vi "Main.vi"(11 "Module Admin":refnum<class "Delacor_lib_QMH_Module Admin.lvclass">) -> ()   [LabVIEW 2024, in "Acquire.lvlib"]
doc: "This template is based off of the Queued Message Handler design pattern and the Queued Message Handler project template that ships with LabVIEW.\n\nThe main difference is that the queue is private to this module and communication between modules is performed via Broadcast and Request events.\n\nRequest events are wrapped in public API methods and are handled in the Event Handling Loop (EHL) of this VI. Any module can register for Broadcast events sent by this module. The EHL generates messages based on user interface actions.\n\nThe Message Handling Loop (MHL) processes messages generated by the EHL, or by other messages. The messages are string values, so new messages can be added easily to the Message Cases case structure in the MHL. Each message cluster can also provide an optional value for Message Data, which is a variant that can be converted to whatever message-specific data is required.\n_____\nBased on DQMH Project Template 7.0.1.1316."
uses:
  Acquire.lvlib
  <vilib>/Delacor/Delacor QMH/Libraries/Module Admin_class/Delacor_lib_QMH_Module Admin.lvclass
  Module Data--cluster.ctl
  <vilib>/Delacor/Delacor QMH/Libraries/Message Queue_class/Delacor_lib_QMH_Message Queue.lvclass/Delacor_lib_QMH_Message Queue.ctl
  Stop Argument--cluster.ctl
  <vilib>/Delacor/Delacor QMH/Libraries/Module Admin_class/Delacor_lib_QMH_Module Admin.lvclass/Delacor_lib_QMH_Module Admin.ctl
  Data Received Argument--cluster.ctl
  Start Recording Argument--cluster.ctl
  Stop Recording Argument--cluster.ctl
  Start Acquisition Argument--cluster.ctl
  Stop Acquisition Argument--cluster.ctl
  Get Reference Argument--cluster.ctl
  Get Reference (Reply Payload)--cluster.ctl
  DAQ/DAQ Config.ctl
  <vilib>/Delacor/Delacor QMH/Libraries/Message Queue_class/Delacor_lib_QMH_Enqueue Message (Single).vi
  <vilib>/Delacor/Delacor QMH/Libraries/Module Admin_class/Delacor_lib_QMH_Get External Launch.vi
  <vilib>/Delacor/Delacor QMH/Libraries/Message Queue_class/Delacor_lib_QMH_Message Queue.lvclass
  DAQ/DAQ.lvlib
panel:
  out "Waveform Chart":waveform(dbl)[](graph)
  in  "Acquire":bool
  in  "Record":bool
  out "error out":errorcluster
  out "Status":string
  in  "Simulate MHL Error":bool
  in  "Simulate EHL Error":bool
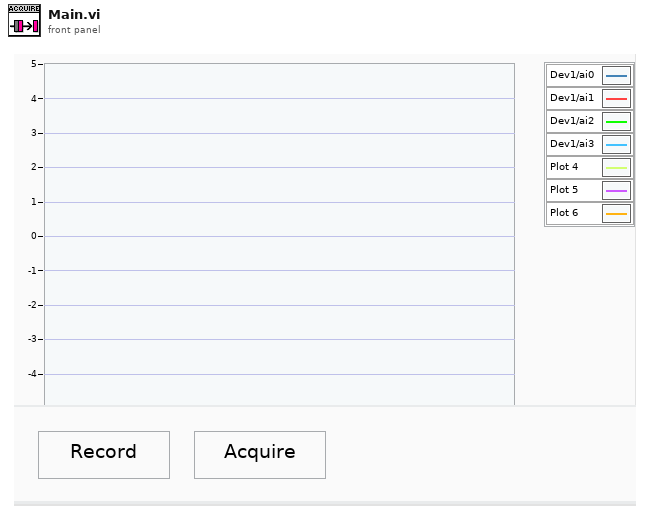
[diagram p1: front panel]
types:
  T1 = typedef "Acquire.lvlib/Request Events--cluster.ctl" = cluster{"Stop Module":refnum<user-event>, "Show Panel":refnum<user-event>, "Hide Panel":refnum<user-event>, "Get Module Execution Status":refnum<user-event>, "Show Diagram":refnum<user-event>, "Private":cluster{"Data Received":refnum<user-event>}, "Start Recording":refnum<user-event>, "Stop Recording":refnum<user-event>, "Start Acquisition":refnum<user-event>, "Stop Acquisition":refnum<user-event>, "Get Reference":refnum<user-event>}
  T2 = typedef "DAQ.lvlib/Broadcast Events--cluster.ctl" = cluster{"Module Did Init":refnum<user-event>, "Status Updated":refnum<user-event>, "Error Reported":refnum<user-event>, "Module Did Stop":refnum<user-event>, "Update Module Execution Status":refnum<user-event>, "New Data":refnum<user-event>}
  T3 = typedef "Acquire.lvlib/Module Data--cluster.ctl" = cluster{"Status":string, "Recording?":bool, "tdms file out":refnum<k34>, "Acquiring?":bool}
  T4 = enum32{"invalid lock state", "Not Locked", "Locked (No Password)", "Password-protected"}
  T5 = typedef "Acquire.lvlib/Stop Argument--cluster.ctl" = cluster{"Origin":string, "Exit via Stop Module Req?":bool, "Wait for Module to stop?":bool}
  T6 = typedef "Acquire.lvlib/Data Received Argument--cluster.ctl" = cluster{"Data":waveform(dbl)[]}
  T7 = typedef "Acquire.lvlib/Start Recording Argument--cluster.ctl" = cluster{"File Path":path}
  T8 = typedef "Acquire.lvlib/Stop Recording Argument--cluster.ctl" = cluster{"Boolean":bool}
  T9 = typedef "Acquire.lvlib/Start Acquisition Argument--cluster.ctl" = cluster{"Boolean":bool}
  T10 = typedef "Acquire.lvlib/Stop Acquisition Argument--cluster.ctl" = cluster{"Boolean":bool}
  T11 = typedef "Acquire.lvlib/Get Reference Argument--cluster.ctl" = cluster{"Wait Notifier":refnum<notifier>, "wait for reply":bool}
  T12 = enum32{"Invalid", "Standard", "Closed", "Hidden", "Minimized", "Maximized"}
  T13 = enum16{"open", "open or create", "create or replace", "create", "open (read-only)"}
  T14 = typedef "DAQ.lvlib/DAQ Config.ctl" = cluster{"DAQmx Channel":tag, "Samplerate":dbl, "# Samples":i32}
  T15 = typedef "Acquire.lvlib/Get Reference (Reply Payload)--cluster.ctl" = cluster{"Main VI":refnum<vi>, "error":errorcluster}
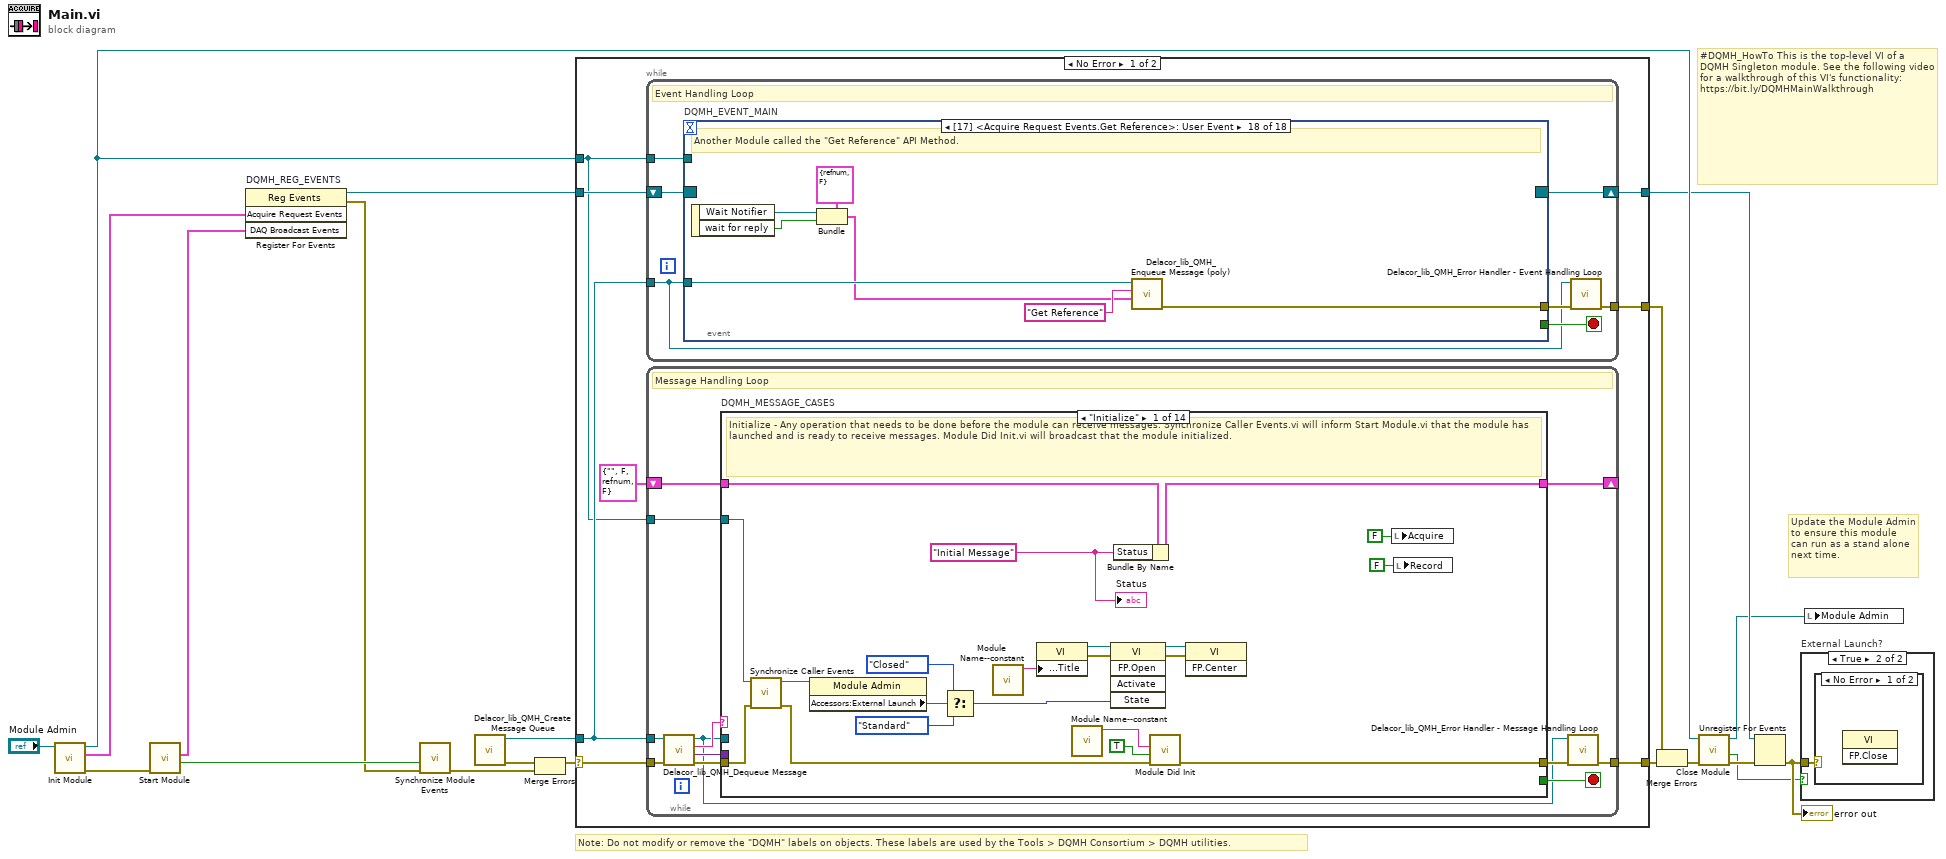
[diagram p0: block diagram]
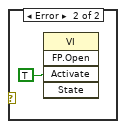
[diagram p3: hidden frame]
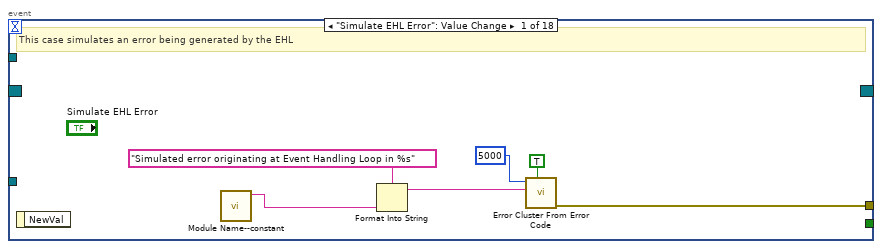
[diagram p4: hidden frame]
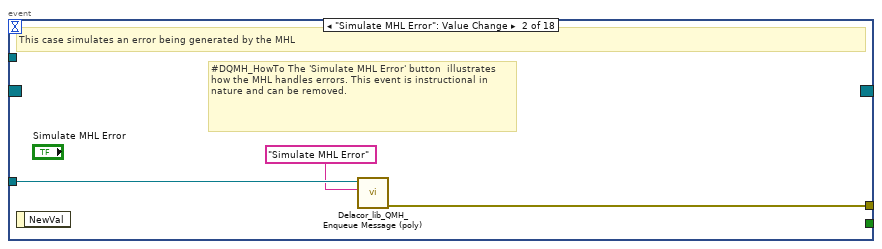
[diagram p5: hidden frame]
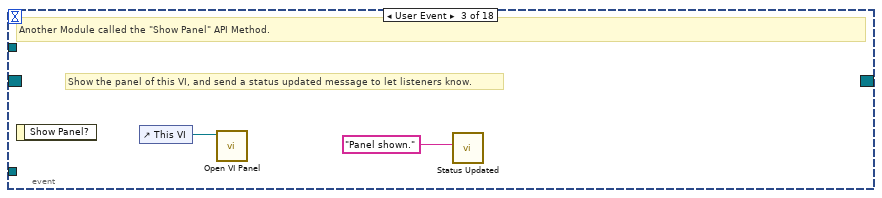
[diagram p6: hidden frame]
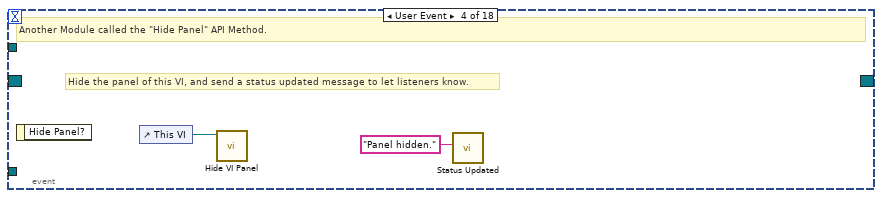
[diagram p7: hidden frame]
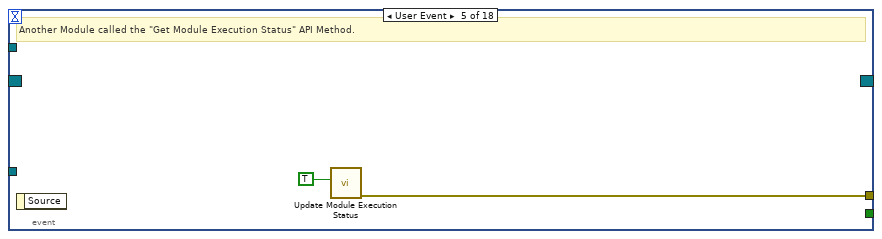
[diagram p8: hidden frame]
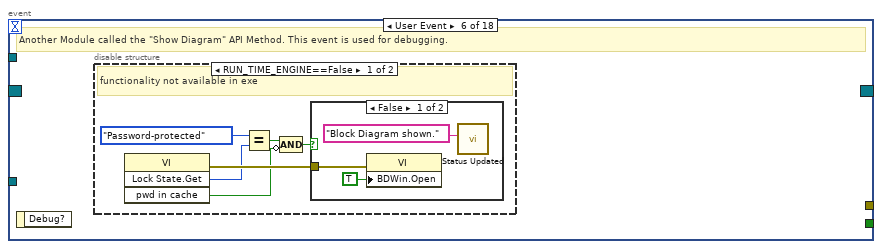
[diagram p9: hidden frame]
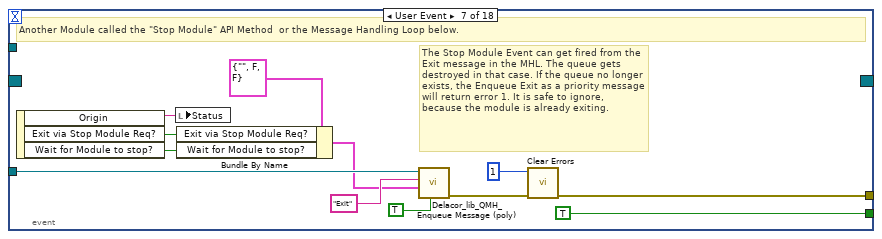
[diagram p12: hidden frame]
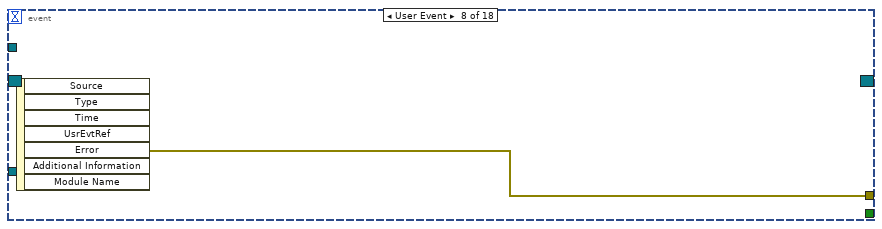
[diagram p13: hidden frame]
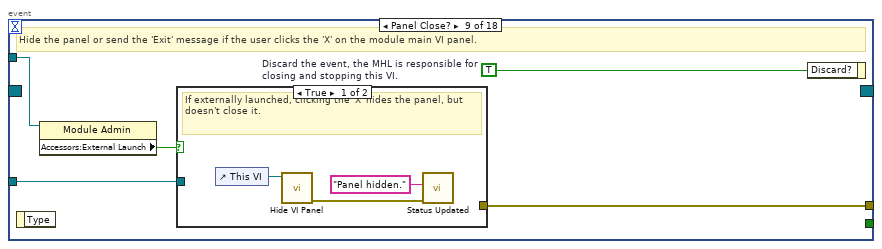
[diagram p14: hidden frame]
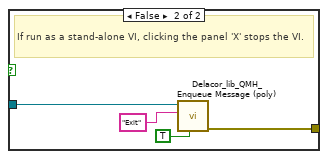
[diagram p15: hidden frame]
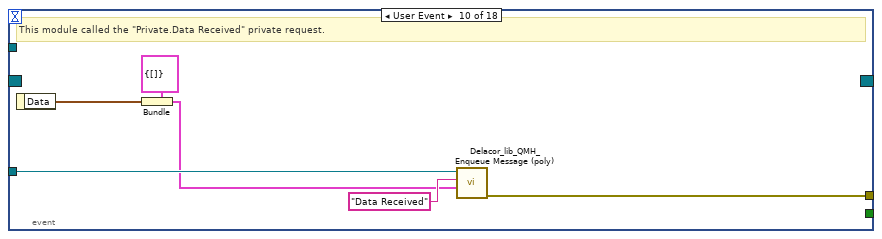
[diagram p16: hidden frame]
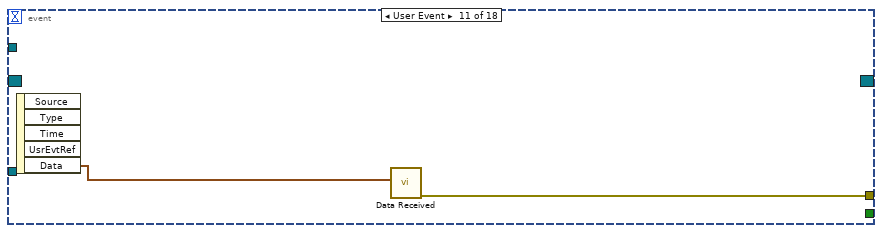
[diagram p17: hidden frame]
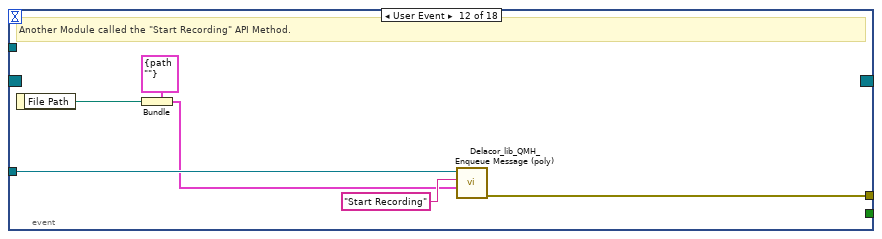
[diagram p18: hidden frame]
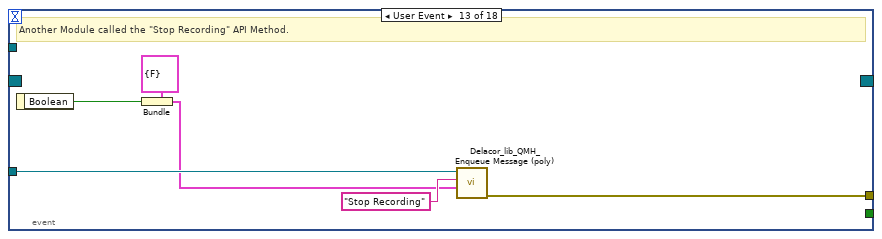
[diagram p19: hidden frame]
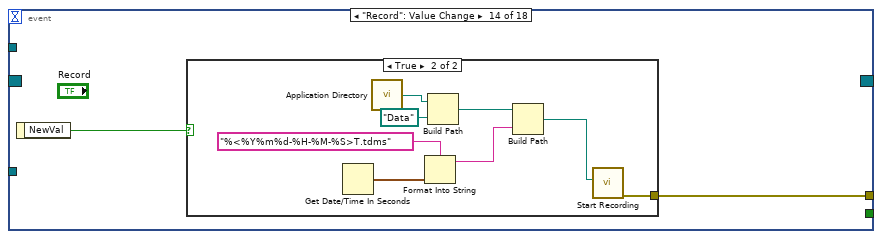
[diagram p20: hidden frame]
diagram:
  # "#DQMH_HowTo This is the top-level VI of a DQMH Singleton module. See the following video for a walkthrough of this VI's functionality: https://bit.ly/DQMHMainWalkthrough"
  # "Note: Do not modify or remove the \"DQMH\" labels on objects. These labels are used by the Tools > DQMH Consortium > DQMH utilities."
  # "Update the Module Admin to ensure this module can run as a stand alone next time."
  n1 = call "Init Module.vi"("Singleton Module Admin in"="Module Admin") -> ("error out"=w19:errorcluster, "Acquire Request Events"=w9:T1, "Singleton Module Admin out"=w12:refnum<class "Delacor_lib_QMH_Module Admin.lvclass">)  [unwired: 8 in]
  n2 = call "Start Module.vi"("error in"=w19) -> ("Wait for Event Sync?"=w3:bool, "DAQ Broadcast Events"=w4:T2)  [unwired: 7 in, 2 out]
  n3 = register-events "DQMH_REG_EVENTS"(w9, w4) -> (reference out=w10:refnum<event-registration>, error out=w2:errorcluster)  [unwired: 2 in]
  n4 = call "Synchronize Module Events.vi"("error in"=w2, "Wait for Event Sync?"=w3) -> ("error out"=w1:errorcluster)  [unwired: 9 in]
  n5 = call <vilib>:"Delacor_lib_QMH_Create Message Queue.vi"() -> ("error out"=w14:errorcluster, "Message Queue"=w8:refnum<class "Delacor_lib_QMH_Message Queue.lvclass">)  [unwired: 10 in]
  n6 = Merge Errors(w14, w1) -> (w13:errorcluster)
  n7 = case shown="No Error" w13 {
    selector: w13 -> [w26 w332]
    tunnel: [w28 w331] -> w20
    tunnel: [w25 w330] -> w11
    tunnel: w10 -> [w23 w330]
    tunnel: w8 -> [w22 w325]
    tunnel: [w27 _] -> w17
    tunnel: w12 -> [w21 w326]
    frame No Error {
      n8 = while {
        tunnel: w22 -> [w29]
        shift-right: [w32] -> w25
        shift-left: w23 -> [w33]
        tunnel: [w34] -> w27
        tunnel: w21 -> [w30]
        stop <- w31 stop-if-true
        # "Event Handling Loop"
        n9 = event "DQMH_EVENT_MAIN" shown="[17] <Acquire Request Events.Get Reference>: User Event" {
          selector: w33 -> [_ _ _ _ _ _ _ _ _ _ _ _ _ _ _ _ _ _]
          dyn-events: [_ _ _ _ _ _ _ _ _ _ _ _ _ _ _ _ _ _] -> w32
          timeout: _ -> [_ _ _ _ _ _ _ _ _ _ _ _ _ _ _ _ _ _]
          tunnel: [_ _ _ _ _ _ TRUE ("Discard?") _ _ _ _ _ _ _ _ _ _ _] -> w31
          tunnel: w29 -> [_ w43 _ _ _ _ w67 _ w75 w90 _ w98 w104 _ _ w125 w131 w138]
          tunnel: [w41 w44 _ _ w50 _ w70 w72 w77 w85 w91 w93 w99 w105 w117 w120 w126 w132] -> w35
          tunnel: w30 -> [_ _ _ _ _ _ _ _ w74 _ _ _ _ _ _ _ _ _]
          event "Simulate EHL Error": Value Change {
            # "This case simulates an error being generated by the EHL"
            n10 = event-data() -> ()  [unwired: 1 in, 1 out]
            n11 = call "Module Name--constant.vi"() -> ("Module Name"=w38:string)  [unwired: 11 in]
            n12 = Format Into String(format string="Simulated error originating at Event Handling Loop in %s", w38) -> (resulting string=w39:string)  [unwired: 2 in, 1 out]
            n13 = call <vilib>:"Error Cluster From Error Code.vi"("show call chain? (False)"=TRUE, "error message (\"\")"=w39, "error code (0)"=5000) -> ("error out"=w41:errorcluster)  [unwired: 6 in]
          }
          event "Simulate MHL Error": Value Change {
            # "#DQMH_HowTo The 'Simulate MHL Error' button  illustrates how the MHL handles errors. This event is instructional in nature and can be removed."
            # "This case simulates an error being generated by the MHL"
            n14 = event-data() -> ()  [unwired: 1 in, 1 out]
            n15 = call-poly <vilib>:"Delacor_lib_QMH_Enqueue Message (poly).vi"("Message"="Simulate MHL Error", "Message Queue in"=w43) -> ("error out"=w44:errorcluster)  [unwired: 8 in, 1 out]
          }
          event User Event {
            # "Show the panel of this VI, and send a status updated message to let listeners know."
            # "Another Module called the \"Show Panel\" API Method."
            n16 = event-data() -> ()  [unwired: 1 in, 1 out]
            n17 = control-ref of="This VI"() -> (w46:refnum<vi>)
            n18 = call "Open VI Panel.vi"("VI"=w46) -> ()  [unwired: 10 in, 1 out]
            n19 = call "Status Updated.vi"("Status"="Panel shown." ("format string")) -> ()  [unwired: 10 in, 1 out]
          }
          event User Event {
            # "Hide the panel of this VI, and send a status updated message to let listeners know."
            # "Another Module called the \"Hide Panel\" API Method."
            n20 = event-data() -> ()  [unwired: 1 in, 1 out]
            n21 = control-ref of="This VI"() -> (w48:refnum<vi>)
            n22 = call "Hide VI Panel.vi"("VI"=w48) -> ()  [unwired: 10 in, 1 out]
            n23 = call "Status Updated.vi"("Status"="Panel hidden." ("format string")) -> ()  [unwired: 10 in, 1 out]
          }
          event User Event {
            # "Another Module called the \"Get Module Execution Status\" API Method."
            n24 = event-data() -> ()  [unwired: 1 in, 1 out]
            n25 = call "Update Module Execution Status.vi"("Running?"=TRUE) -> ("error out"=w50:errorcluster)  [unwired: 10 in]
          }
          event User Event {
            # "Another Module called the \"Show Diagram\" API Method. This event is used for debugging."
            n26 = event-data() -> ()  [unwired: 1 in, 1 out]
            n27 = disable-structure shown="RUN_TIME_ENGINE==False" {
              frame condition #0 (active) {
                # "functionality not available in exe"
                n28 = invoke on="Invoke Node" class="VI" method="Lock State.Get"() -> (error out=w56:errorcluster, "Get Lock State"=w55:T4, "pwd in cache"=w52:bool)  [unwired: 4 in, 1 out]
                n29 = Equal?(x=T4."Password-protected", y=w55) -> (x = y?=w53:bool)
                n30 = Compound Arithmetic op=AND(w53, invert w52) -> (w51:bool)
                n31 = case shown="False" w51 {
                  tunnel: w56 -> [w59 _]
                  frame False {
                    n32 = property on="Property Node" class="VI"(error in=w59, "BDWin.Open"=TRUE ("Block Diagram Window:Open")) -> ()  [unwired: 1 in, 2 out]
                    n33 = call "Status Updated.vi"("Status"="Block Diagram shown." ("format string")) -> ()  [unwired: 10 in, 1 out]
                  }
                  frame True {
                    # "Password-protected VI, and the password is not in the cache. Do not show the diagram."
                  }
                }
              }
              frame condition #1 {
              }
            }
          }
          event User Event {
            # "The Stop Module Event can get fired from the Exit message in the MHL. The queue gets destroyed in that case. If the queue no longer exists, the Enqueue Exit as a priority message will return error 1. It is safe to ignore, because the module is already exiting."
            # "Another Module called the \"Stop Module\" API Method  or the Message Handling Loop below."
            n34 = event-data() -> ("Origin"=w66:string, "Exit via Stop Module Req?"=w62:bool, "Wait for Module to stop?"=w61:bool)  [unwired: 1 in]
            n35 = local write "Status"(w66) -> ()
            n36 = Bundle By Name(cluster=T5 {"Origin"="", "Exit via Stop Module Req?"=FALSE, "Wait for Module to stop?"=FALSE} ("Stop Argument"), "Exit via Stop Module Req?"=w62, "Wait for Module to stop?"=w61) -> (w60:T5)
            n37 = call-poly <vilib>:"Delacor_lib_QMH_Enqueue Message (poly).vi"("Priority Message? (F)"=TRUE, "Message Data"=w60, "Message"="Exit", "Message Queue in"=w67) -> ("error out"=w71:errorcluster)  [unwired: 6 in, 1 out]
            n38 = call <vilib>:"Clear Errors.vi"("error in (no error)"=w71, "specific error code to clear (0: all)"=1) -> ("error out"=w70:errorcluster)  [unwired: 4 in, 1 out]
          }
          event User Event {
            n39 = event-data() -> ("Error"=w72:errorcluster)  [unwired: 1 in, 6 out]
          }
          event Panel Close? {
            w76 = TRUE  # Discard the event, the MHL is responsible for closing and stopping this VI.
            # "Hide the panel or send the 'Exit' message if the user clicks the 'X' on the module main VI panel."
            n40 = event-data() -> ()  [unwired: 1 in, 1 out]
            n41 = property on="Property Node" class="Module Admin"(reference=w74) -> ("Accessors:External Launch"=w73:bool)  [unwired: 1 in, 2 out]
            n42 = case shown="True" w73 {
              tunnel: w75 -> [_ w83]
              tunnel: [_ w84] -> w77
              frame True {
                # "If externally launched, clicking the 'X' hides the panel, but doesn't close it."
                n43 = control-ref of="This VI"() -> (w80:refnum<vi>)
                n44 = call "Hide VI Panel.vi"("VI"=w80) -> ("error out"=w78:errorcluster)  [unwired: 10 in]
                n45 = call "Status Updated.vi"("error in"=w78, "Status"="Panel hidden." ("format string")) -> ()  [unwired: 9 in, 1 out]
              }
              frame False {
                # "If run as a stand-alone VI, clicking the panel 'X' stops the VI."
                n46 = call-poly <vilib>:"Delacor_lib_QMH_Enqueue Message (poly).vi"("Priority Message? (F)"=TRUE, "Message"="Exit", "Message Queue in"=w83) -> ("error out"=w84:errorcluster)  [unwired: 7 in, 1 out]
              }
            }
            n47 = event-data ("Event Filter Node")("Discard?"=w76) -> ()  [unwired: 1 in, 1 out]
          }
          event User Event {
            # "This module called the \"Private.Data Received\" private request."
            n48 = event-data() -> ("Data"=w86:waveform(dbl)[])  [unwired: 1 in]
            n49 = Bundle(cluster=T6 {"Data"=[]} ("Data Received Argument"), "Data"=w86) -> (w87:T6)
            n50 = call-poly <vilib>:"Delacor_lib_QMH_Enqueue Message (poly).vi"("Message Data"=w87, "Message"="Data Received", "Message Queue in"=w90) -> ("error out"=w85:errorcluster)  [unwired: 7 in, 1 out]
          }
          event User Event {
            n51 = event-data() -> ("Data"=w92:waveform(dbl)[])  [unwired: 1 in, 4 out]
            n52 = call "Data Received.vi"("Data"=w92) -> ("error out"=w91:errorcluster)  [unwired: 10 in]
          }
          event User Event {
            # "Another Module called the \"Start Recording\" API Method."
            n53 = event-data() -> ("File Path"=w94:path)  [unwired: 1 in]
            n54 = Bundle(cluster=T7 {"File Path"=path ""} ("Start Recording Argument"), "File Path"=w94) -> (w95:T7)
            n55 = call-poly <vilib>:"Delacor_lib_QMH_Enqueue Message (poly).vi"("Message Data"=w95, "Message"="Start Recording", "Message Queue in"=w98) -> ("error out"=w93:errorcluster)  [unwired: 7 in, 1 out]
          }
          event User Event {
            # "Another Module called the \"Stop Recording\" API Method."
            n56 = event-data() -> ("Boolean"=w100:bool)  [unwired: 1 in]
            n57 = Bundle(cluster=T8 {"Boolean"=FALSE} ("Stop Recording Argument"), "Boolean"=w100) -> (w101:T8)
            n58 = call-poly <vilib>:"Delacor_lib_QMH_Enqueue Message (poly).vi"("Message Data"=w101, "Message"="Stop Recording", "Message Queue in"=w104) -> ("error out"=w99:errorcluster)  [unwired: 7 in, 1 out]
          }
          event "Record": Value Change {
            n59 = event-data() -> ("NewVal"=w106:bool)  [unwired: 1 in]
            n60 = case shown="True" w106 {
              tunnel: [w107 w115] -> w105
              frame False {
                n61 = call "Stop Recording.vi"() -> ("error out"=w107:errorcluster)  [unwired: 11 in]
              }
              frame True {
                n62 = Get Date/Time In Seconds() -> (seconds since 1Jan1904=w112:timestamp)
                n63 = call <vilib>:"Application Directory.vi"() -> ("Application Directory"=w109:path)
                n64 = Format Into String(format string="%<%Y%m%d-%H-%M-%S>T.tdms", w112) -> (resulting string=w114:string)  [unwired: 2 in, 1 out]
                n65 = Build Path(base path=w109, name or relative path=path "Data") -> (appended path=w111:path)
                n66 = Build Path(base path=w111, name or relative path=w114) -> (appended path=w108:path)
                n67 = call "Start Recording.vi"("File Path"=w108) -> ("error out"=w115:errorcluster)  [unwired: 10 in]
              }
            }
          }
          event "Acquire": Value Change {
            n68 = event-data() -> ("NewVal"=w116:bool)  [unwired: 1 in]
            n69 = case shown="True" w116 {
              tunnel: [w118 w119] -> w117
              frame False {
                n70 = call "Stop Acquisition.vi"() -> ("error out"=w118:errorcluster)  [unwired: 11 in]
              }
              frame True {
                n71 = call "Start Acquisition.vi"() -> ("error out"=w119:errorcluster)  [unwired: 11 in]
              }
            }
          }
          event User Event {
            # "Another Module called the \"Start Acquisition\" API Method."
            n72 = event-data() -> ("Boolean"=w121:bool)  [unwired: 1 in]
            n73 = Bundle(cluster=T9 {"Boolean"=FALSE} ("Start Acquisition Argument"), "Boolean"=w121) -> (w122:T9)
            n74 = call-poly <vilib>:"Delacor_lib_QMH_Enqueue Message (poly).vi"("Message Data"=w122, "Message"="Start Acquisition", "Message Queue in"=w125) -> ("error out"=w120:errorcluster)  [unwired: 7 in, 1 out]
          }
          event User Event {
            # "Another Module called the \"Stop Acquisition\" API Method."
            n75 = event-data() -> ("Boolean"=w127:bool)  [unwired: 1 in]
            n76 = Bundle(cluster=T10 {"Boolean"=FALSE} ("Stop Acquisition Argument"), "Boolean"=w127) -> (w128:T10)
            n77 = call-poly <vilib>:"Delacor_lib_QMH_Enqueue Message (poly).vi"("Message Data"=w128, "Message"="Stop Acquisition", "Message Queue in"=w131) -> ("error out"=w126:errorcluster)  [unwired: 7 in, 1 out]
          }
          event User Event {
            # "Another Module called the \"Get Reference\" API Method."
            n78 = event-data() -> ("Wait Notifier"=w134:refnum<notifier>, "wait for reply"=w133:bool)  [unwired: 1 in]
            n79 = Bundle(cluster=T11 {"Wait Notifier"=refnum, "wait for reply"=FALSE} ("Get Reference Argument"), "Wait Notifier"=w134, "wait for reply"=w133) -> (w135:T11)
            n80 = call-poly <vilib>:"Delacor_lib_QMH_Enqueue Message (poly).vi"("Message Data"=w135, "Message"="Get Reference", "Message Queue in"=w138) -> ("error out"=w132:errorcluster)  [unwired: 7 in, 1 out]
          }
        }
        n81 = call-dynamic "Delacor_lib_QMH_Error Handler - Event Handling Loop.vi"("error in"=w35, "Message Queue in"=w29) -> ("dup error in"=w34:errorcluster)  [unwired: 8 in, 1 out]
      }
      n82 = while {
        tunnel: w22 -> [w139]
        shift-right: [w147] -> _
        shift-left: T3 {"Status"="", "Recording?"=FALSE, "tdms file out"=refnum, "Acquiring?"=FALSE} ("Data Cluster") -> [w148]
        tunnel: w26 -> [w150]
        tunnel: [w142] -> w28
        tunnel: w21 -> [w143]
        stop <- w146 stop-if-true
        # "Message Handling Loop"
        n83 = call-dynamic "Delacor_lib_QMH_Dequeue Message.vi"("error in"=w150, "Message Queue in"=w139) -> ("error out"=w149:errorcluster, "Message Data"=w144:variant, "Message"=w145:string, "Message Queue out"=w140:refnum<class "Delacor_lib_QMH_Message Queue.lvclass">)  [unwired: 6 in]
        n84 = case "DQMH_MESSAGE_CASES" shown="\"Initialize\"" w145 {
          selector: w145 -> [_ _ _ _ _ _ _ _ _ _ _ _ _ w320]
          tunnel: w140 -> [_ _ _ _ _ _ _ _ _ _ _ w285 w308 _]
          tunnel: w149 -> [w169 w173 w185 w204 w231 w244 w252 w265 w270 w272 w281 w292 w314 w323]
          tunnel: [w167 w173 w180 w198 w229 w245 w251 w255 w269 w272 w280 w288 w309 w324] -> w141
          tunnel: w148 -> [w158 w172 w178 w196 w228 w248 w253 w264 w268 w271 w278 w287 w307 w321]
          tunnel: [w157 w172 w177 w199 w230 w243 w250 w264 w268 w271 w278 w287 w307 w321] -> w147
          tunnel: [_ _ _ _ _ _ _ _ _ _ _ _ w306 _] -> w146
          tunnel: w144 -> [_ _ w183 w202 _ _ _ w262 _ _ _ w286 w305 _]
          tunnel: w143 -> [w159 _ _ _ _ _ _ _ _ _ _ w284 w300 _]
          frame "Initialize" {
            w153 = "Initial Message" ("Initial Message")
            # "Initialize - Any operation that needs to be done before the module can receive messages. Synchronize Caller Events.vi will inform Start Module.vi that the module has launched and is ready to receive messages. Module Did Init.vi will broadcast that the module initialized."
            n85 = call "Synchronize Caller Events.vi"("error in"=w169, "Singleton Module Admin in"=w159) -> ("error out"=w168:errorcluster, "Singleton Module Admin out"=w154:refnum<class "Delacor_lib_QMH_Module Admin.lvclass">)  [unwired: 8 in]
            n86 = property on="Property Node" class="Module Admin"(reference=w154) -> ("Accessors:External Launch"=w163:bool)  [unwired: 1 in, 2 out]
            n87 = Select(t=T12."Closed" ("State"), s=w163, f=T12."Standard" ("State")) -> (s? t:f=w160:T12)
            n88 = call "Module Name--constant.vi"() -> ("Module Name"=w166:string)  [unwired: 11 in]
            n89 = property on="Property Node" class="VI"("Front Panel.Title"=w166) -> (reference out=w165:refnum<vi>, error out=w171:errorcluster)  [unwired: 2 in]
            n90 = call "Module Name--constant.vi"() -> ("Module Name"=w155:string)  [unwired: 11 in]
            n91 = invoke on="Invoke Node" class="VI" method="FP.Open"(reference=w165, error in=w171, "State"=w160) -> (reference out=w164:refnum<vi>, error out=w170:errorcluster)  [unwired: 2 in, 3 out]
            n92 = Bundle By Name(cluster=w158, "Status"=w153) -> (w157:T3)
            n93 = call "Module Did Init.vi"("error in"=w168, "Initialized?"=TRUE, "Origin"=w155) -> ("error out"=w167:errorcluster)  [unwired: 8 in]
            n94 = invoke on="Invoke Node" class="VI" method="FP.Center"(reference=w164, error in=w170) -> ()  [unwired: 1 in, 3 out]
            n95 = local write "Acquire"(FALSE ("Acquire")) -> ()
            n96 = local write "Record"(FALSE ("Record")) -> ()
            "Status" <- w153
          }
          frame "---Module Specific---" {
            # "Separator -- The following cases handle messages specific to this Module."
          }
          frame "Data Received" {
            # "New data received from DAQ module."
            n97 = Variant To Data(error in=w185, type=T6 {"Data"=[]} ("Data Received Argument"), Variant=w183) -> (data=w181:T6, error out=w184:errorcluster)
            n98 = Unbundle By Name(w181) -> ("Data"=w179:waveform(dbl)[])
            "Waveform Chart" <- w179
            n99 = Unbundle By Name(w178) -> ("Recording?"=w174:bool, "tdms file out"=w176:refnum<k34>)
            n100 = case shown="True" w174 {
              tunnel: w184 -> [w186 w192]
              tunnel: [w186 w191] -> w180
              tunnel: w179 -> [_ w190]
              tunnel: w176 -> [w187 w189]
              tunnel: [w187 w188] -> w175
              frame False {
              }
              frame True {
                n101 = TDMS Write(0:w189, 9:w190, 11:w192) -> (4:w188:refnum<k34>, 15:w191:errorcluster)  [unwired: 3 in, 2 out]
              }
            }
            n102 = Bundle By Name(cluster=w178, "tdms file out"=w175) -> (w177:T3)
          }
          frame "Start Recording" {
            # "Starts logging received data to a file."
            n103 = Variant To Data(error in=w204, type=T7 {"File Path"=path ""} ("Start Recording Argument"), Variant=w202) -> (data=w200:T7, error out=w203:errorcluster)
            n104 = Unbundle By Name(w196) -> ("Recording?"=w195:bool, "Acquiring?"=w193:bool)
            n105 = Unbundle By Name(w200) -> ("File Path"=w197:path)
            n106 = Compound Arithmetic op=AND(invert w195, w193) -> (w194:bool)
            n107 = case shown="True" w194 {
              tunnel: w196 -> [w208 w226]
              tunnel: w203 -> [w206 w225]
              tunnel: [w208 w224] -> w199
              tunnel: [w205 w220] -> w198
              tunnel: w197 -> [_ w217]
              tunnel: w193 -> [w207 _]
              frame False {
                n108 = case shown="True" w207 {
                  tunnel: [w210 w213] -> w205
                  tunnel: w206 -> [w211 w214]
                  frame False {
                    n109 = call "Status Updated.vi"("error in"=w211, "Status"="Warning: Start Acquisition before Recording") -> ("error out"=w210:errorcluster)  [unwired: 9 in]
                  }
                  frame True {
                    n110 = call "Status Updated.vi"("error in"=w214, "Status"="Warning: Recording already in progress") -> ("error out"=w213:errorcluster)  [unwired: 9 in]
                  }
                }
              }
              frame True {
                n111 = TDMS Open(8:w225, 10:T13."create or replace" ("operation (0:open)"), 11:w217) -> (0:w222:errorcluster, 3:w221:refnum<k34>)  [unwired: 4 in]
                n112 = Bundle By Name(cluster=w226, "Recording?"=TRUE ("Logging?"), "tdms file out"=w221) -> (w224:T3)
                n113 = Strip Path(path=w217) -> (name=w216:string)  [unwired: 1 out]
                n114 = Format Into String(format string="Recording to file %s started." ("Status"), w216) -> (resulting string=w218:string)  [unwired: 2 in, 1 out]
                n115 = call "Status Updated.vi"("error in"=w222, "Status"=w218) -> ("error out"=w220:errorcluster)  [unwired: 9 in]
              }
            }
          }
          frame "Stop Recording" {
            # "Stops writing to tdms and closes the file."
            n116 = Unbundle By Name(w228) -> ("Recording?"=w227:bool)
            n117 = case shown="True" w227 {
              tunnel: w231 -> [w234 w241]
              tunnel: [w235 w240] -> w230
              tunnel: w228 -> [w235 w238]
              tunnel: [w233 w237] -> w229
              frame False {
                n118 = call "Status Updated.vi"("error in"=w234, "Status"="Warning: Not Recording") -> ("error out"=w233:errorcluster)  [unwired: 9 in]
              }
              frame True {
                n119 = Unbundle By Name(w238) -> ("tdms file out"=w236:refnum<k34>)
                n120 = Bundle By Name(cluster=w238, "Recording?"=FALSE ("Logging?")) -> (w240:T3)
                n121 = TDMS Close(8:w241, 11:w236) -> (0:w237:errorcluster)  [unwired: 1 out]
              }
            }
          }
          frame "Start Acquisition" {
            # "Starts an Aquisition in the DAQ module."
            n122 = Bundle By Name(cluster=w248, "Acquiring?"=TRUE) -> (w243:T3)
            n123 = call "Configure Acquisition.vi"("error in"=w244, "DAQ Config"=T14 {"DAQmx Channel"="Dev1/ai0:3", "Samplerate"=1000.0, "# Samples"=100}) -> ("error out"=w246:errorcluster)  [unwired: 9 in]
            n124 = call "Start Acquisition.vi"("error in"=w246) -> ("error out"=w245:errorcluster)  [unwired: 10 in]
          }
          frame "Stop Acquisition" {
            # "Stops the acquisition in the DAQ Module."
            n125 = Bundle By Name(cluster=w253, "Acquiring?"=FALSE) -> (w250:T3)
            n126 = call "Stop Acquisition.vi"("error in"=w252) -> ("error out"=w251:errorcluster)  [unwired: 10 in]
          }
          frame "Get Reference" {
            # "Returns the main.vi reference to insert it into a subpanel of a calling VI."
            n127 = Variant To Data(error in=w265, type=T11 {"Wait Notifier"=refnum, "wait for reply"=FALSE} ("Get Reference Argument"), Variant=w262) -> (data=w260:T11, error out=w263:errorcluster)
            n128 = Unbundle By Name(w260) -> ("Wait Notifier"=w259:refnum<notifier>, "wait for reply"=w258:bool)
            n129 = control-ref of="This VI"() -> (w254:refnum<vi>)
            n130 = Bundle By Name(cluster=T15 {"Main VI"=refnum, "error"={"status"=FALSE, "code"=0, "source"=""}} ("Get Reference (Reply Payload)"), "Main VI"=w254) -> (w257:T15)
            n131 = Merge Errors(w263) -> (w255:errorcluster)
            n132 = case "DQMH_FIRE_NOTIFIER" shown="True" w258 {
              tunnel: w259 -> [_ w267]
              tunnel: w257 -> [_ w266]
              frame False {
              }
              frame True {
                n133 = Send Notification(notification=w266, notifier=w267) -> ()  [unwired: 1 in, 2 out]
              }
            }
          }
          frame "---Copy This Frame---" {
            # "Duplicate this frame when creating new messages.  Change this comment in the duplicated frame to describe this message."
            n134 = Merge Errors(w270) -> (w269:errorcluster)
          }
          frame "---Exit and Error Handling---" {
            # "Separator - The following cases handle errors and exit messages."
          }
          frame "Simulate MHL Error" {
            # "#DQMH_HowTo The 'Simulate MHL Error' button  illustrates how the MHL handles errors. This event is instructional in nature and can be removed."
            # "Simulate an error occurring at the MHL"
            n135 = call "Module Name--constant.vi"() -> ("Module Name"=w274:string)  [unwired: 11 in]
            n136 = Format Into String(format string="Simulated error originating at Message Handling Loop in %s", w274) -> (resulting string=w275:string)  [unwired: 2 in, 1 out]
            n137 = call <vilib>:"Error Cluster From Error Code.vi"("show call chain? (False)"=TRUE, "error message (\"\")"=w275, "error code (0)"=5001) -> ("error out"=w279:errorcluster)  [unwired: 6 in]
            n138 = Merge Errors(w281, w279) -> (w280:errorcluster)
          }
          frame "Error" {
            # "#CodeRecommended - If the module is running in standalone mode (External Launch = FALSE), this code will pop up an error dialog and call the 'Exit' message if an error occurs. Add more fine-grained error management here."
            # "Error - Check the error message data and respond accordingly. This message is sent by the \"Error Handler\" VIs at the end of each loop in this application."
            n139 = property on="Property Node" class="Module Admin"(reference=w284) -> ("Accessors:External Launch"=w283:bool)  [unwired: 1 in, 2 out]
            n140 = Variant To Data(error in=w292, type=errorcluster {"status"=FALSE, "code"=0, "source"=""} ("error constant"), Variant=w286) -> (data=w282:errorcluster, error out=w290:errorcluster)
            n141 = local write "error out"(w282) -> ()
            n142 = call "Error Reported.vi"("Error"=w282) -> ()  [unwired: 10 in, 1 out]
            n143 = case shown="False" w283 {
              tunnel: [w297 _] -> w289
              tunnel: w285 -> [w295 _]
              tunnel: w282 -> [w296 _]
              frame False {
                n144 = disable-structure shown="Default" {
                  disable-tunnel: w296 -> [w298 _]
                  frame condition #0 (active) {
                    # "If the module is running standalone, then pop up an error dialog and call the \"Exit\" message."
                    n145 = call <vilib>:"Simple Error Handler.vi"("error in (no error)"=w298) -> ()  [unwired: 4 in, 5 out]
                  }
                  frame condition #1 {
                    # "To prevent the Simple Error Handler VI from being loaded (e.g. when deploying to a Real-Time target), add the Conditional Disable Symbol \"DQMH_Disable_SEH\" to your project and set it to TRUE."
                  }
                }
                n146 = call-poly <vilib>:"Delacor_lib_QMH_Enqueue Message (poly).vi"("Priority Message? (F)"=TRUE, "Message"="Exit", "Message Queue in"=w295) -> ("error out"=w297:errorcluster)  [unwired: 7 in, 1 out]
              }
              frame True {
                # "If the module was launched externally, calling the Error Reported broadcast VI is the only action performed by the \"Error\" message. The module's caller can then process the error appropriately."
              }
            }
            n147 = Merge Errors(w290, w289) -> (w288:errorcluster)
          }
          frame "Exit" {
            w304 = 91  # 91: not all Exit messages will have an argument
            w306 = TRUE  # Stop the VI
            # "Release the message queue reference"
            # "Exit - Exit the application."
            n148 = Variant To Data(error in=w314, type=T5 {"Origin"="", "Exit via Stop Module Req?"=FALSE, "Wait for Module to stop?"=FALSE} ("Stop Argument"), Variant=w305) -> (data=w302:T5, error out=w311:errorcluster)
            n149 = call <vilib>:"Clear Errors.vi"("error in (no error)"=w311, "specific error code to clear (0: all)"=w304) -> ("error out"=w313:errorcluster)  [unwired: 4 in, 1 out]
            n150 = call "Stop Module.vi"("error in"=w313) -> ("error out"=w299:errorcluster)  [unwired: 10 in]
            n151 = control-ref of="This VI"() -> (w301:refnum<vi>)
            n152 = call-dynamic "Delacor_lib_QMH_Release Message Queue.vi"("error in"=w299, "Message Queue"=w308) -> ("error out"=w312:errorcluster)  [unwired: 9 in]
            n153 = call "Handle Exit.vi"("Stop Argument"=w302, "Admin in"=w300, "VI reference"=w301) -> ("error out"=w310:errorcluster)  [unwired: 7 in, 1 out]
            n154 = Merge Errors(w312, w310) -> (w309:errorcluster)
            n155 = call "Error Reported.vi"("Error"=w309) -> ()  [unwired: 10 in, 1 out]
          }
          frame Default {
            # "'Default' case only runs if there is a message that isn't defined in any of the other cases.  Output a programming error."
            n156 = call "Module Name--constant.vi"() -> ("Module Name"=w319:string)  [unwired: 11 in]
            n157 = Format Into String(format string="The invalid message string \"%s\" was received in the Message Handling Loop for module \"%s\".", w320, w319) -> (resulting string=w315:string)  [unwired: 2 in, 1 out]
            n158 = call <vilib>:"Error Cluster From Error Code.vi"("show call chain? (False)"=TRUE, "error message (\"\")"=w315, "error code (0)"=1) -> ("error out"=w322:errorcluster)  [unwired: 6 in]
            n159 = Merge Errors(w323, w322) -> (w324:errorcluster)
          }
        }
        n160 = call-dynamic "Delacor_lib_QMH_Error Handler - Message Handling Loop.vi"("error in"=w141, "Message Queue in"=w140) -> ("dup error in"=w142:errorcluster)  [unwired: 8 in, 1 out]
      }
    }
    frame Error {
      # "Synchronize Caller Events.vi will inform Start Module.vi that the module has launched and will let the code calling Start Module.vi register for broadcasts and would permit the caller receive the broadcast that an error occurred at launch time."
      n161 = call-dynamic "Delacor_lib_QMH_Release Message Queue.vi"("error in"=w332, "Message Queue"=w325) -> ("error out"=w331:errorcluster)  [unwired: 9 in]
      n162 = call "Synchronize Caller Events.vi"("Singleton Module Admin in"=w326) -> ("error out"=w333:errorcluster)  [unwired: 9 in, 1 out]
      n163 = call "Module Name--constant.vi"() -> ("Module Name"=w329:string)  [unwired: 11 in]
      n164 = Format Into String(format string="An error occurred during initialization. %s is no longer running.", w329) -> (resulting string=w327:string)  [unwired: 2 in, 1 out]
      n165 = Merge Errors(w331, w333) -> (w334:errorcluster)
      n166 = call "Error Reported.vi"("Additional Information"=w327, "Error"=w334) -> ()  [unwired: 9 in, 1 out]
    }
  }
  n167 = Merge Errors(w17, w20) -> (w16:errorcluster)
  n168 = call "Close Module.vi"("error in"=w16, "Module Admin in"=w12) -> ("error out"=w18:errorcluster, "External Launch"=w5:bool, "Module Admin out"=w6:refnum<class "Delacor_lib_QMH_Module Admin.lvclass">)  [unwired: 7 in]
  n169 = Unregister For Events(event registration refnum=w11, error in=w18) -> (error out=w15:errorcluster)
  "error out" <- w15
  n170 = case "External Launch?" shown="True" w5 {
    tunnel: w15 -> [_ w335]
    frame False {
    }
    frame True {
      n171 = case shown="No Error" w335 {
        frame No Error {
          n172 = invoke on="Invoke Node" class="VI" method="FP.Close"() -> ()  [unwired: 3 in, 3 out]
        }
        frame Error {
          n173 = invoke on="Invoke Node" class="VI" method="FP.Open"("Activate"=TRUE ("Activate?")) -> ()  [unwired: 4 in, 5 out]
        }
      }
    }
  }
  n174 = local write "Module Admin"(w6) -> ()
